vi "MGI Parse Format String.vi"(8 "error in (no error)":errorcluster, 9 "Offset in":i32, 11 "String":string="Hello %#4_1g\nas time:\n%<%H:%M:%S%> %m>t") -> (0 "error out":errorcluster, 1 "Offset out":i32, 2 "Delim":string, 3 "FormatCode":T1)   [LabVIEW 2020]
doc: "Parses the string at the specified position for a format code. The portion of the string before the format code is output as \"Delim\". If an error occurs, then an error is output and the Offset out is -1.\n\nAuthored by Shawn Walpole\nsupport@mooregoodideas.com\nwww.mooregoodideas.com\n\nCopyright (c) 2010, Moore Good Ideas, Inc.\n\nAll rights reserved.\n\nRedistribution and use in source and binary forms, with or without modification, are permitted provided that the following conditions are met:\n\n * Redistributions of source code must retain the above copyright notice, this list of conditions and the following disclaimer.\n * Redistributions in binary form must reproduce the above copyright notice, this list of conditions and the following disclaimer in the documentation and/or other materials provided with the distribution.\n * Neither the name of Moore Good Ideas, Inc. nor the names of its contributors may be used to endorse or promote products derived from this software without specific prior written permission.\n\nTHIS SOFTWARE IS PROVIDED BY THE COPYRIGHT HOLDERS AND CONTRIBUTORS \"AS IS\" AND ANY EXPRESS OR IMPLIED WARRANTIES, INCLUDING, BUT NOT LIMITED TO, THE IMPLIED WARRANTIES OF MERCHANTABILITY AND FITNESS FOR A PARTICULAR PURPOSE ARE DISCLAIMED. IN NO EVENT SHALL THE COPYRIGHT OWNER OR CONTRIBUTORS BE LIABLE FOR ANY DIRECT, INDIRECT, INCIDENTAL, SPECIAL, EXEMPLARY, OR CONSEQUENTIAL DAMAGES (INCLUDING, BUT NOT LIMITED TO, PROCUREMENT OF SUBSTITUTE GOODS OR SERVICES; LOSS OF USE, DATA, OR PROFITS; OR BUSINESS INTERRUPTION) HOWEVER CAUSED AND ON ANY THEORY OF LIABILITY, WHETHER IN CONTRACT, STRICT LIABILITY, OR TORT (INCLUDING NEGLIGENCE OR OTHERWISE) ARISING IN ANY WAY OUT OF THE USE OF THIS SOFTWARE, EVEN IF ADVISED OF THE POSSIBILITY OF SUCH DAMAGE."
uses:
  <userlib>/_MGI/String/MGI Format String Code Cluster.ctl
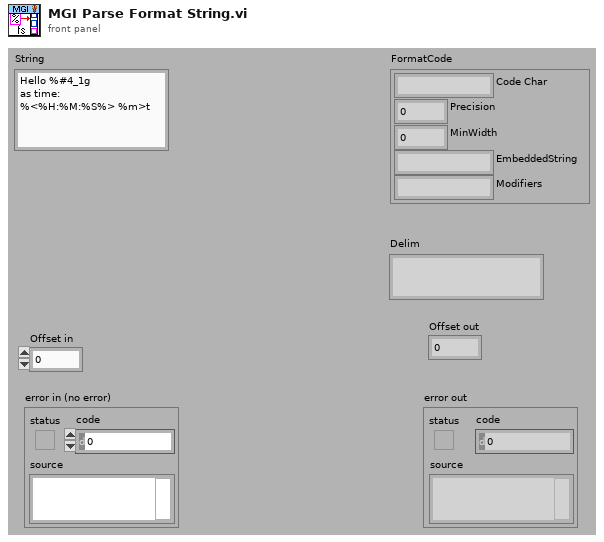
[diagram p1: front panel]
types:
  T1 = typedef "MGI Format String Code Cluster.ctl" = cluster{"Code Char":string, "Precision":i32, "MinWidth":i32, "EmbeddedString":string, "Modifiers":string}
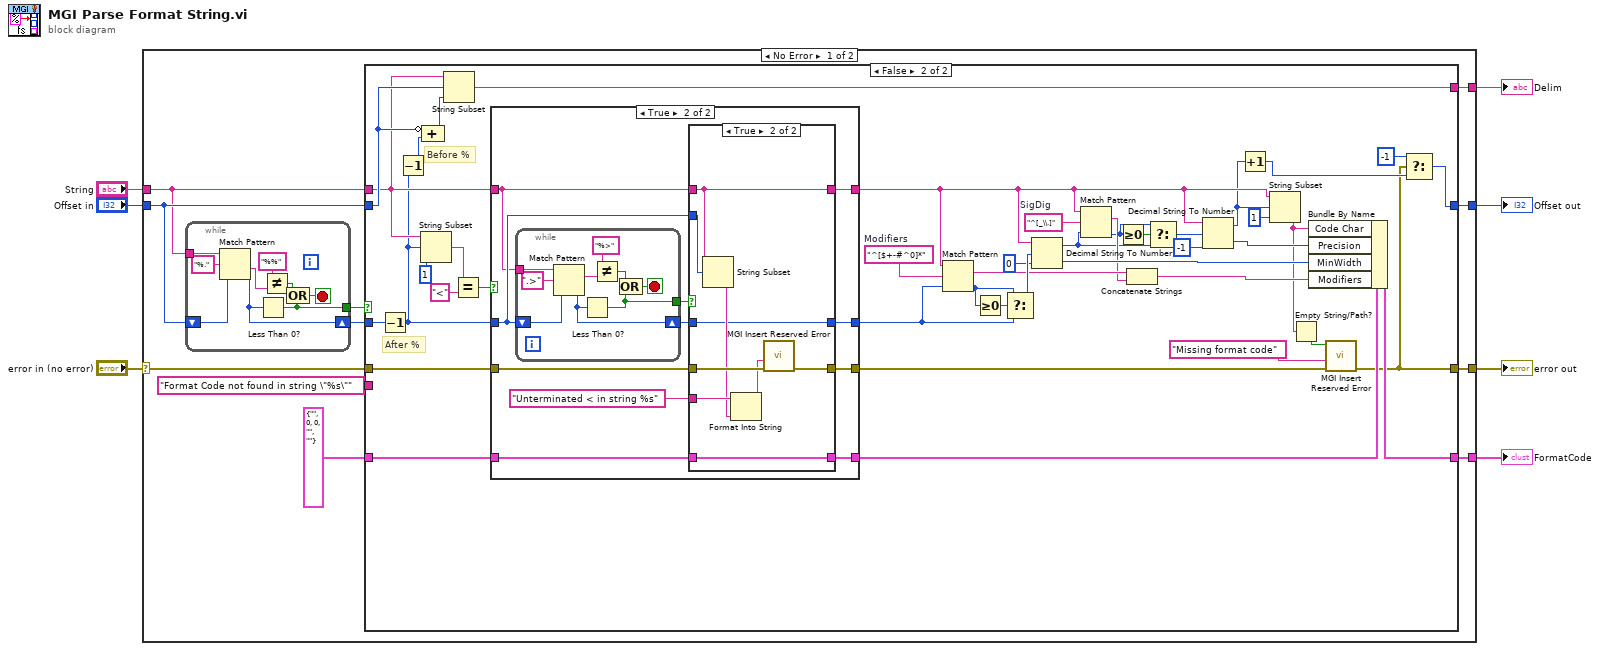
[diagram p0: block diagram]
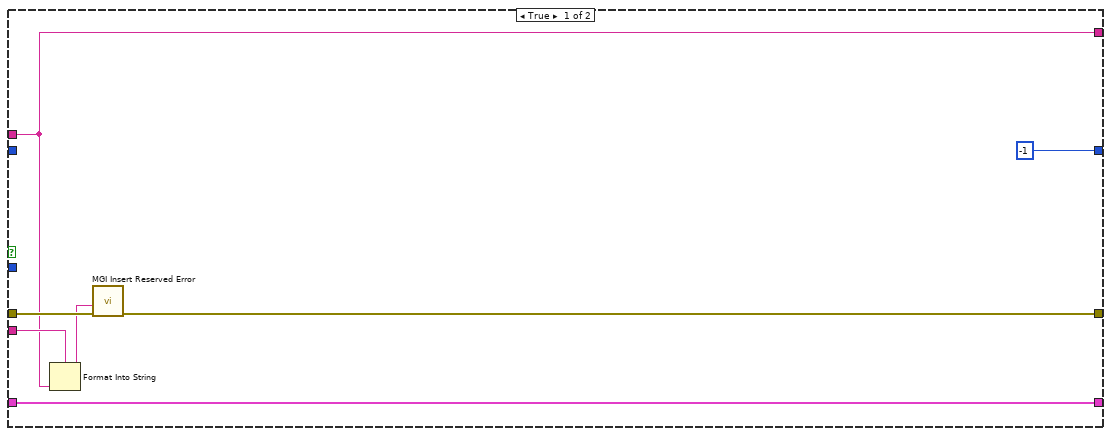
[diagram p2: hidden frame]
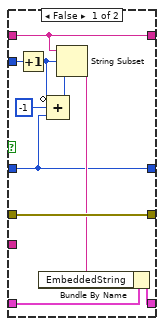
[diagram p4: hidden frame]
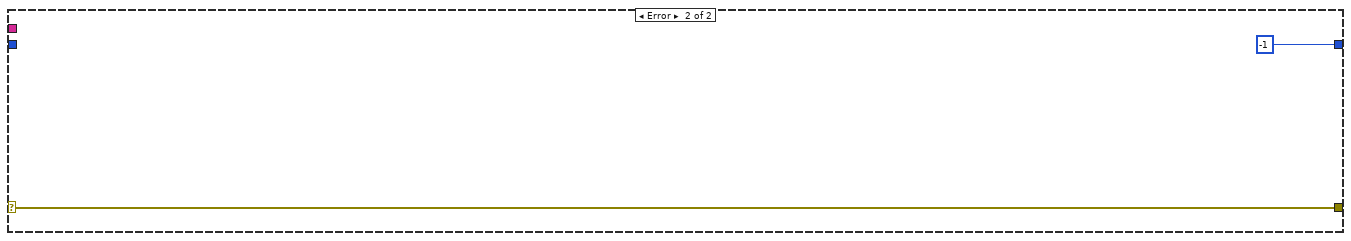
[diagram p5: hidden frame]
diagram:
  n1 = case shown="No Error" "error in (no error)" {
    selector: "error in (no error)" -> [w18 w122]
    tunnel: "String" -> [w12 _]
    tunnel: [w16 _] -> w6
    tunnel: [w9 w122] -> w2
    tunnel: "Offset in" -> [w15 _]
    tunnel: [w10 _] -> w3
    tunnel: [w8 -1 ("Offset in")] -> w1
    frame No Error {
      n2 = while {
        tunnel: w12 -> [w120]
        shift-right: [w114] -> w14
        shift-left: w15 -> [w119]
        tunnel: [w112] -> w13
        stop <- w113 stop-if-true
        n3 = Match Pattern(string=w120, regular expression="%.", offset (0)=w119) -> (after substring=w117:string, offset past match=w114:i32)  [unwired: 2 out]
        n4 = Less Than 0?(x=w114) -> (x < 0?=w112:bool)
        n5 = Not Equal?(x="%%" ("regular expression"), y=w117) -> (x != y?=w115:bool)
        n6 = Compound Arithmetic op=OR(w115, w112) -> (w113:bool)
      }
      n7 = case shown="False" w13 {
        tunnel: w18 -> [w25 w57]
        tunnel: "Format Code not found in string \"%s\"" ("Error Description") -> [w24 _]
        tunnel: [w22 w68] -> w16
        tunnel: w15 -> [_ w66]
        tunnel: w14 -> [_ w65]
        tunnel: w12 -> [w22 w59]
        tunnel: T1 {"Code Char"="", "Precision"=0, "MinWidth"=0, "EmbeddedString"="", "Modifiers"=""} ("FormatCode") -> [w21 w56]
        tunnel: [w21 w35] -> w10
        tunnel: [w20 w28] -> w9
        tunnel: [-1 w26] -> w8
        frame True {
          n8 = Format Into String(format string=w24, w22) -> (resulting string=w23:string)  [unwired: 2 in, 1 out]
          n9 = call <userlib>:"MGI Insert Reserved Error.vi"("Error In"=w25, "Error Description"=w23) -> ("Error Out"=w20:errorcluster)  [unwired: 9 in]
        }
        frame False {
          w54 = "^[$+-#^0]*"  # Modifiers
          w48 = "^[_\\.]"  # SigDig
          # "After %"
          # "Before %"
          n10 = Decrement(x=w65) -> (x-1=w58:i32)
          n11 = Decrement(x=w58) -> (x-1=w64:i32)
          n12 = String Subset(string=w59, offset (0)=w58, length (rest)=1 ("length (rest)")) -> (substring=w62:string)
          n13 = Compound Arithmetic op=ADD(invert w66, w64) -> (w67:i32)
          n14 = String Subset(string=w59, offset (0)=w66, length (rest)=w67) -> (substring=w68:string)
          n15 = Equal?(x=w62, y="<") -> (x = y?=w60:bool)
          n16 = case shown="True" w60 {
            tunnel: w59 -> [w72 w80]
            tunnel: w58 -> [w69 w81]
            tunnel: w57 -> [w70 w83]
            tunnel: [w72 w77] -> w37
            tunnel: [w70 w78] -> w33
            tunnel: w56 -> [w71 w75]
            tunnel: [w71 w74] -> w55
            tunnel: [w69 w73] -> w52
            frame False {
            }
            frame True {
              n17 = while {
                tunnel: w80 -> [w111]
                shift-right: [w108] -> w76
                shift-left: w81 -> [w110]
                tunnel: [w103] -> w79
                stop <- w107 stop-if-true
                n18 = Match Pattern(string=w111, regular expression=".>", offset (0)=w110) -> (match substring=w106:string, offset past match=w108:i32)  [unwired: 2 out]
                n19 = Less Than 0?(x=w108) -> (x < 0?=w103:bool)
                n20 = Not Equal?(x="%>", y=w106) -> (x != y?=w105:bool)
                n21 = Compound Arithmetic op=OR(w105, w103) -> (w107:bool)
              }
              n22 = case shown="True" w79 {
                tunnel: w83 -> [w88 w102]
                tunnel: "Unterminated < in string %s" ("Error Description") -> [_ w101]
                tunnel: w81 -> [w92 w97]
                tunnel: w80 -> [w93 w98]
                tunnel: [w88 w99] -> w78
                tunnel: [w93 w98] -> w77
                tunnel: w76 -> [w84 w94]
                tunnel: w75 -> [w87 w95]
                tunnel: [w85 w95] -> w74
                tunnel: [w84 w94] -> w73
                frame False {
                  n23 = Increment(x=w92) -> (x+1=w91:i32)
                  n24 = Compound Arithmetic op=ADD(invert w91, -1 ("value"), w84) -> (w90:i32)
                  n25 = String Subset(string=w93, offset (0)=w91, length (rest)=w90) -> (substring=w86:string)
                  n26 = Bundle By Name(cluster=w87, "EmbeddedString"=w86) -> (w85:T1)
                }
                frame True {
                  n27 = String Subset(string=w98, offset (0)=w97) -> (substring=w96:string)  [unwired: 1 in]
                  n28 = Format Into String(format string=w101, w96) -> (resulting string=w100:string)  [unwired: 2 in, 1 out]
                  n29 = call <userlib>:"MGI Insert Reserved Error.vi"("Error In"=w102, "Error Description"=w100) -> ("Error Out"=w99:errorcluster)  [unwired: 9 in]
                }
              }
            }
          }
          n30 = Match Pattern(string=w37, regular expression=w54, offset (0)=w52) -> (match substring=w45:string, offset past match=w51:i32)  [unwired: 2 out]
          n31 = Greater Or Equal To 0?(x=w51) -> (x >= 0?=w53:bool)
          n32 = Select(t=w51, s=w53, f=w52) -> (s? t:f=w50:i32)
          n33 = Decimal String To Number(string=w37, offset=w50, default (0L)=0 ("default (0 I32)")) -> (offset past number=w42:i32, number=w47:i32)
          n34 = Match Pattern(string=w37, regular expression=w48, offset (0)=w42) -> (match substring=w44:string, offset past match=w41:i32)  [unwired: 2 out]
          n35 = Greater Or Equal To 0?(x=w41) -> (x >= 0?=w46:bool)
          n36 = Concatenate Strings(w45, w44) -> (w43:string)
          n37 = Select(t=w41, s=w46, f=w42) -> (s? t:f=w40:i32)
          n38 = Decimal String To Number(string=w37, offset=w40, default (0L)=-1 ("default (0 I32)")) -> (offset past number=w34:i32, number=w38:i32)
          n39 = Increment(x=w34) -> (x+1=w29:i32)
          n40 = String Subset(string=w37, offset (0)=w34, length (rest)=1 ("length (rest)")) -> (substring=w31:string)
          n41 = Empty String/Path?(string/path=w31) -> (empty?=w32:bool)
          n42 = Bundle By Name(cluster=w55, "Code Char"=w31, "Precision"=w38, "MinWidth"=w47, "Modifiers"=w43) -> (w35:T1)
          n43 = call <userlib>:"MGI Insert Reserved Error.vi"("Error In"=w33, "Error Description"="Missing format code", "Error? (T)"=w32) -> ("Error Out"=w28:errorcluster)  [unwired: 8 in]
          n44 = Select(t=-1, s=w28, f=w29) -> (s? t:f=w26:i32)
        }
      }
    }
    frame Error {
    }
  }
  "Delim" <- w6
  "FormatCode" <- w3
  "error out" <- w2
  "Offset out" <- w1
